vi "Double Exponential Decay Fit.vi"(8 "Peak Value":dbl, 10 "Y":dbl[](array[numeric]), 11 "X":dbl[](array[numeric])) -> (0 "f(X,a)":dbl[](array[numeric]), 1 "residue":dbl, 2 "Parameter Names":string[](array[string]), 3 "best fit parameters":dbl[](array[numeric]))   [LabVIEW 2022 SP3]
doc: "This demonstrates how to use nonlinear curve fitting to fit an ellipse. \nThis problem is modelled as a 2D curve fit (2 domains, 1 range), \nwhere the X and Y data are the noisy points, and Z is 1."
uses:
  <vilib>/gmath/NumericalOptimization/Nonlinear Curve Fit LM bound.vi
  <vilib>/gmath/NI_Gmath.lvlib
panel:
  out "Average Timeconstant":dbl
  out "XY Graph":cluster{"X":dbl[], "f(X,a)":dbl[]}[](graph)
  out "#function calls":i32
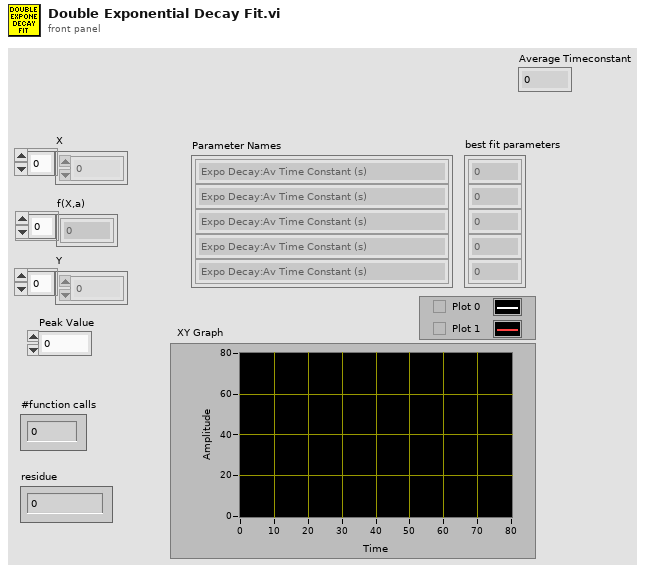
[diagram p1: front panel]
types:
  T1 = cluster{"parameter minimum":dbl[], "parameter maximum":dbl[]}
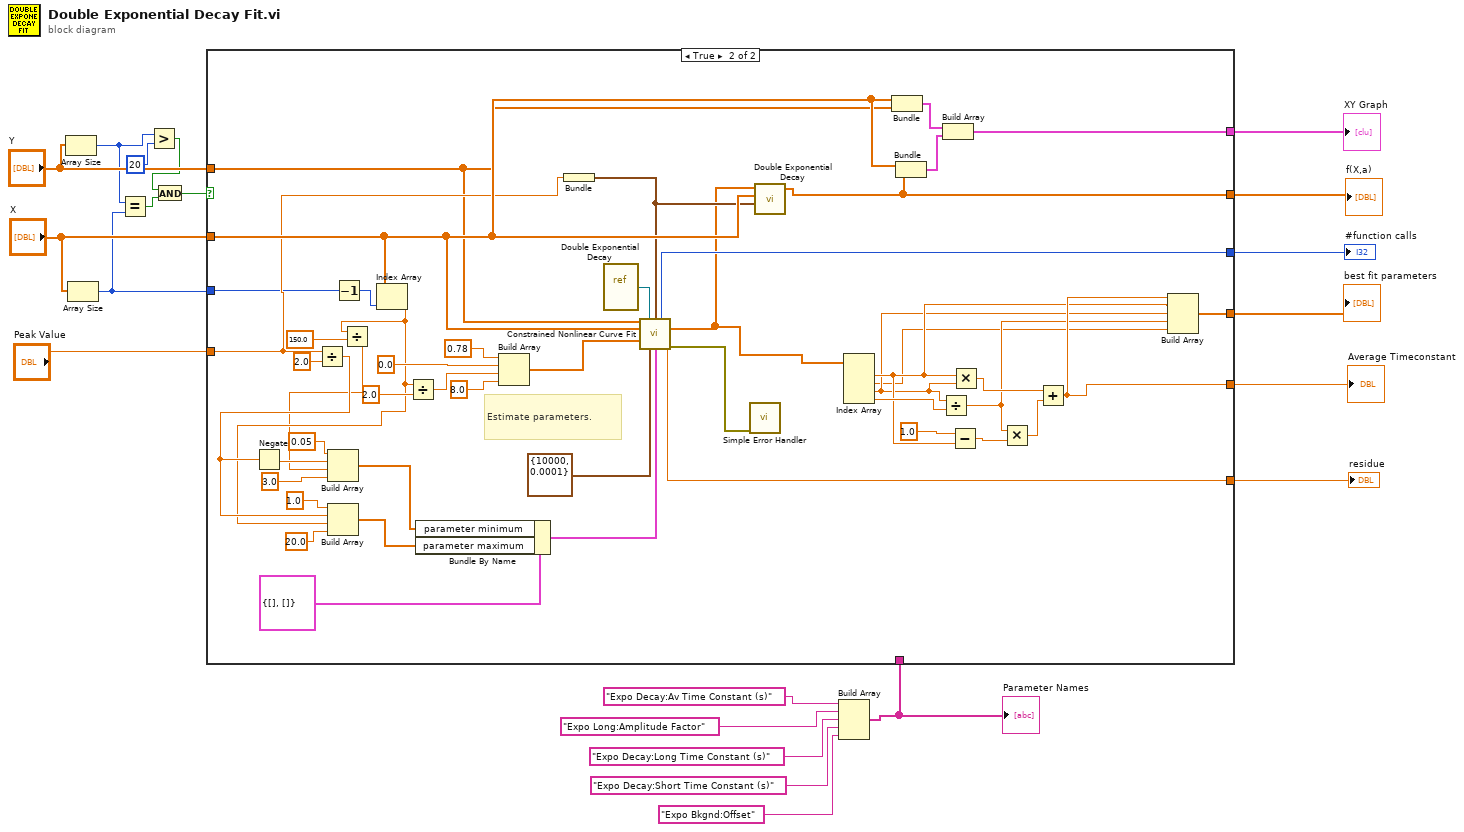
[diagram p0: block diagram]
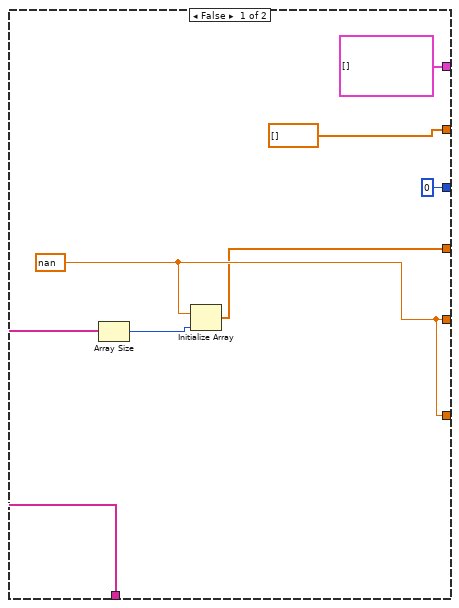
[diagram p2: hidden frame]
diagram:
  n1 = Array Size(array="Y") -> (size(s)=w11:i32)
  n2 = Array Size(array="X") -> (size(s)=w12:i32)
  n3 = Equal?(x=w11, y=w12) -> (x = y?=w9:bool)
  n4 = Greater?(x=w11, y=20) -> (0:w8:bool)
  n5 = And(x=w8, y=w9) -> (x .and. y?=w2:bool)
  n6 = Build Array("Expo Decay:Av Time Constant (s)", "Expo Long:Amplitude Factor", "Expo Decay:Long Time Constant (s)", "Expo Decay:Short Time Constant (s)", "Expo Bkgnd:Offset") -> (w1:string[])
  "Parameter Names" <- w1
  n7 = case shown="True" w2 {
    tunnel: [w24 w74] -> w21
    tunnel: [0 ("number of function calls") w72] -> w20
    tunnel: "X" -> [_ w65]
    tunnel: [dbl[] [] ("f(X,a)") w64] -> w18
    tunnel: [cluster{"X":dbl[], "f(X,a)":dbl[]}[] [] w61] -> w17
    tunnel: "Peak Value" -> [_ w59]
    tunnel: [w24 w40] -> w15
    tunnel: [w22 w38] -> w14
    tunnel: "Y" -> [_ w30]
    tunnel: w12 -> [_ w29]
    tunnel: w1 -> [w26 _]
    frame False {
      w24 = nan
      n8 = Array Size(array=w26) -> (size(s)=w25:i32)
      n9 = Initialize Array(w24, w25) -> (w22:dbl[])
    }
    frame True {
      # "Estimate parameters."
      n10 = Divide(x=w59, y=2.0) -> (x/y=w47:dbl)
      n11 = Negate(x=w47) -> (-x=w48:dbl)
      n12 = Decrement(x=w29) -> (x-1=w68:i32)
      n13 = Index Array(array=w65, index=w68) -> (element=w33:dbl)
      n14 = Build Array(1.0 ("element"), w47, w33, 20.0 ("element")) -> (w49:dbl[])
      n15 = Divide(x=w33, y=150.0) -> (x/y=w31:dbl)
      n16 = Build Array(0.05 ("element"), w48, w31, 3.0 ("element")) -> (w51:dbl[])
      n17 = Divide(x=w33, y=2.0) -> (x/y=w66:dbl)
      n18 = Bundle By Name(cluster=T1 {"parameter minimum"=[], "parameter maximum"=[]} ("parameter bounds"), "parameter minimum"=w51, "parameter maximum"=w49) -> (w46:T1)
      n19 = Build Array(0.78 ("element"), 0.0 ("element"), w66, 8.0 ("element")) -> (w73:dbl[])
      n20 = Bundle("Peak Value"=w59) -> (w57:cluster{"Peak Value":dbl})  [unwired: 1 in]
      n21 = vi-ref "Double Exponential Decay.vi"() -> (w71:refnum<vi>)
      n22 = call-poly <vilib>:"Constrained Nonlinear Curve Fit.vi"("Y"=w30, "f(x,a)"=w71, "data"=w57, "X"=w65, "initial parameters"=w73, "termination"=cluster{"max iteration":i32, "tolerance":dbl} {"max iteration"=10000, "tolerance"=0.0001}, "parameter bounds"=w46) -> ("number of function calls"=w72:i32, "best fit parameters"=w39:dbl[], "residue"=w74:dbl, "error out"=w70:errorcluster)  [unwired: 3 in, 2 out]
      n23 = call <vilib>:"Simple Error Handler.vi"("error in (no error)"=w70) -> ()  [unwired: 4 in, 5 out]
      n24 = call "Double Exponential Decay.vi"("data"=w57, "X"=w65, "a"=w39) -> ("f(X,a)"=w64:dbl[])  [unwired: 1 in, 2 out]
      n25 = Index Array(array=w39) -> (element #1=w37:dbl, element #2=w34:dbl, element #3=w36:dbl, element #4=w42:dbl)  [unwired: 4 in]
      n26 = Bundle("X"=w65, "Y"=w30) -> (w62:cluster{"X":dbl[], "Y":dbl[]})  [unwired: 1 in]
      n27 = Bundle("X"=w65, "f(X,a)"=w64) -> (w63:cluster{"X":dbl[], "f(X,a)":dbl[]})  [unwired: 1 in]
      n28 = Divide(x=w36, y=w42) -> (x/y=w35:dbl)
      n29 = Build Array(w62, w63) -> (w61:cluster{"X":dbl[], "f(X,a)":dbl[]}[])
      n30 = Subtract(x=1.0, y=w37) -> (x-y=w55:dbl)
      n31 = Multiply(x=w37, y=w36) -> (x*y=w53:dbl)
      n32 = Multiply(x=w35, y=w55) -> (x*y=w54:dbl)
      n33 = Add(x=w53, y=w54) -> (x+y=w40:dbl)
      n34 = Build Array(w40, w37, w36, w35, w34) -> (w38:dbl[])
    }
  }
  "residue" <- w21
  "#function calls" <- w20
  "best fit parameters" <- w14
  "XY Graph" <- w17
  "Average Timeconstant" <- w15
  "f(X,a)" <- w18
